vi "snapImg.vi"(1 "Handle in":u32) -> (0 "16bitImgFile":u16[][](array[numeric]))   [LabVIEW 2015]
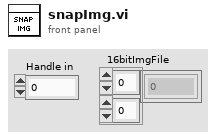
[diagram p1: front panel]
types:
  T1 = cluster{"height":u32, "width":u32, "datatype":u32}
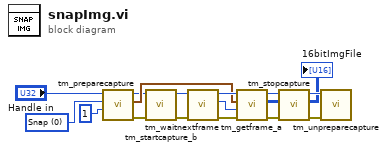
[diagram p0: block diagram]
diagram:
  w2 = 0 items=["Snap", "Sequence"] ("Capture mode")
  n1 = call <userlib>:"tm_preparecapture.vi"("Frames"=1, "Capture mode"=w2, "Handle in"="Handle in") -> ("error out"=w5:errorcluster, "Buffer Info"=w9:T1, "Handle out"=w6:u32)  [unwired: 5 in, 1 out]
  n2 = call <userlib>:"tm_startcapture_b.vi"("error in (no error)"=w5, "Handle in"=w6) -> ("error out"=w8:errorcluster, "Handle out"=w7:u32)  [unwired: 8 in]
  n3 = call <userlib>:"tm_waitnextframe.vi"("error in (no error)"=w8, "Handle in"=w7) -> ("error out"=w11:errorcluster, "Frame Index"=w12:i32, "Handle out"=w10:u32)  [unwired: 6 in, 1 out]
  n4 = call <userlib>:"tm_getframe_a.vi"("error in (no error)"=w11, "Frame Index"=w12, "Buffer Info"=w9, "Handle in"=w10) -> ("error out"=w14:errorcluster, "Data 16"=→"16bitImgFile":u16[][], "Handle out"=w13:u32)  [unwired: 3 in, 2 out]
  n5 = call <userlib>:"tm_stopcapture.vi"("error in (no error)"=w14, "Handle in"=w13) -> ("error out"=w16:errorcluster, "Handle out"=w15:u32)  [unwired: 8 in]
  n6 = call <userlib>:"tm_unpreparecapture.vi"("error in (no error)"=w16, "Handle in"=w15) -> ()  [unwired: 8 in, 2 out]
